vi "data in.vi"() -> ()   [LabVIEW 2017]
panel:
  out "error out 2":errorcluster
  in  "stop":bool
  out "error out":errorcluster
  in  "mode (standard)":T1(ring)
  in  "bytes to read":i32
  out "data out":string
  in  "Send Button":bool
  in  "Port":u16
  in  "address":string
  in  "data in":string
  out "bytes written":i32
  in  "stop 1":bool
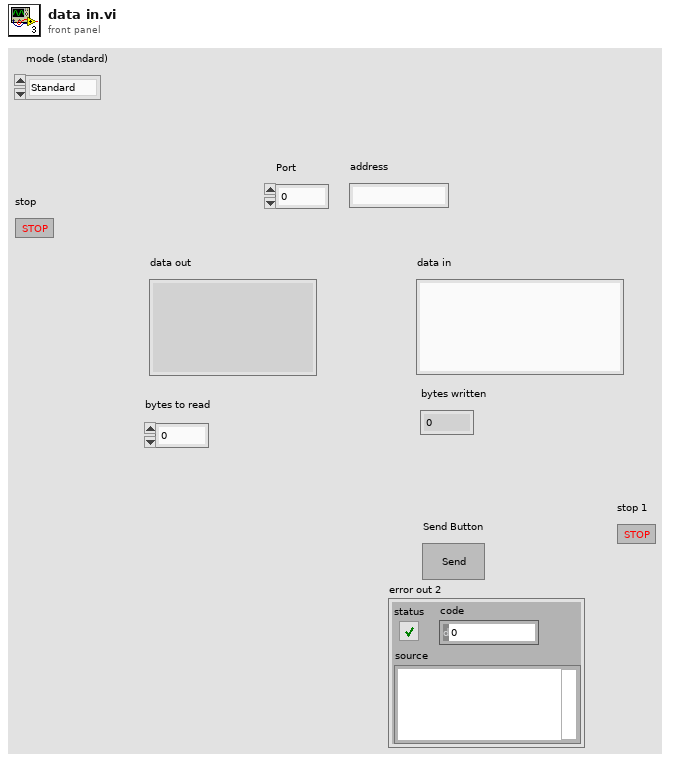
[diagram p1: front panel]
types:
  T1 = enum16{"Standard", "Buffered", "CRLF", "Immediate"}
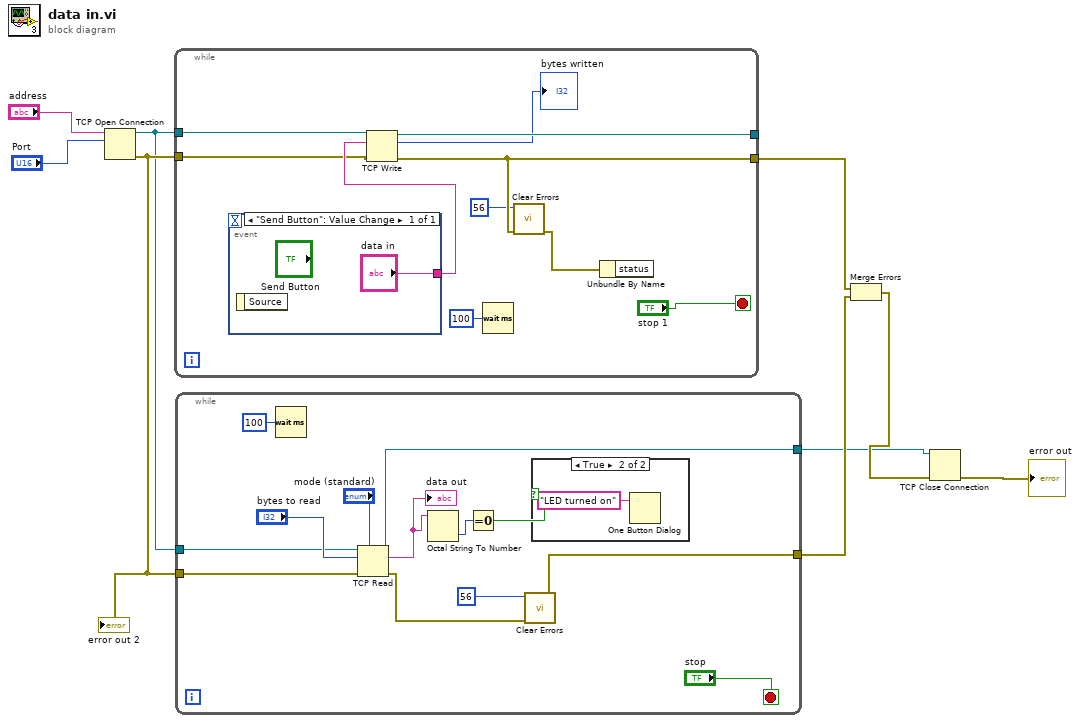
[diagram p0: block diagram]
diagram:
  n1 = TCP Open Connection(address="address", remote port or service name="Port") -> (connection ID=w1:refnum<k5>, error out=w2:errorcluster)  [unwired: 3 in]
  "error out 2" <- w2
  n2 = while {
    tunnel: w1 -> [w16]
    tunnel: [w19] -> _
    tunnel: w2 -> [w15]
    tunnel: [w14] -> w7
    stop <- "stop 1" stop-if-true
    n3 = event shown="[0] \"Send Button\": Value Change" {
      selector: _ -> [_]
      dyn-events: _ -> [_]
      timeout: _ -> [_]
      tunnel: ["data in"] -> w17
      event "Send Button": Value Change {
        n4 = event-data() -> ()  [unwired: 1 in, 1 out]
      }
    }
    n5 = TCP Write(connection ID=w16, data in=w17, error in (no error)=w15) -> (connection ID out=w19:refnum<k5>, bytes written=→"bytes written":i32, error out=w14:errorcluster)  [unwired: 1 in]
    n6 = Wait (ms)(milliseconds to wait=u32 100) -> ()  [unwired: 1 out]
    n7 = call <vilib>:"Clear Errors.vi"("error in (no error)"=w14, "specific error code to clear (0: all)"=56) -> ("error out"=w12:errorcluster)  [unwired: 4 in, 1 out]
    n8 = Unbundle By Name(w12) -> ()  [unwired: 1 out]
  }
  n9 = while {
    tunnel: [w29] -> w4
    tunnel: [w28] -> w3
    tunnel: w2 -> [w27]
    tunnel: w1 -> [w26]
    stop <- "stop" stop-if-true
    n10 = Wait (ms)(milliseconds to wait=u32 100) -> ()  [unwired: 1 out]
    n11 = TCP Read(connection ID=w26, bytes to read="bytes to read", error in (no error)=w27, 7:"mode (standard)") -> (connection ID out=w28:refnum<k5>, data out=w22:string, error out=w32:errorcluster)  [unwired: 1 in]
    "data out" <- w22
    n12 = Octal String To Number(4:w22) -> (0:w21:u32)  [unwired: 2 in, 1 out]
    n13 = Equal To 0?(x=w21) -> (x = 0?=w23:bool)
    n14 = call <vilib>:"Clear Errors.vi"("error in (no error)"=w32, "specific error code to clear (0: all)"=56) -> ("error out"=w29:errorcluster)  [unwired: 4 in, 1 out]
    n15 = case shown="True" w23 {
      frame False {
      }
      frame True {
        n16 = One Button Dialog(message="LED turned on") -> ()  [unwired: 1 in, 1 out]
      }
    }
  }
  n17 = Merge Errors(w7, w4) -> (w6:errorcluster)
  n18 = TCP Close Connection(connection ID=w3, error in (no error)=w6) -> (error out=→"error out":errorcluster)  [unwired: 1 in, 1 out]
